vi "extract-value.vi"(1 "Variable":string, 2 "Chaine contenant valeur":string) -> (0 "Valeur":ext)   [LabVIEW 2018]
panel:
  out "String":string
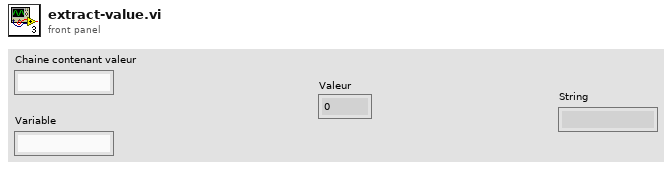
[diagram p1: front panel]
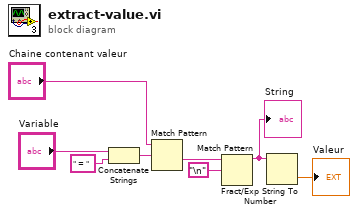
[diagram p0: block diagram]
diagram:
  n1 = Concatenate Strings("Variable", " = " ("regular expression")) -> (w4:string)
  n2 = Match Pattern(string="Chaine contenant valeur", regular expression=w4) -> (after substring=w8:string)  [unwired: 1 in, 3 out]
  n3 = Match Pattern(string=w8, regular expression="\n") -> (before substring=w2:string)  [unwired: 1 in, 3 out]
  "String" <- w2
  n4 = Fract/Exp String To Number(string=w2) -> (number=→"Valeur":dbl)  [unwired: 3 in, 1 out]
